vi "MGI Bezier Time.vi"(1 "t":sgl format="%.2f", 2 "First k":i32, 3 "Bezier Control Points[k]":sgl[](array[numeric]) format="%.4f") -> (0 "u":sgl format="%.2f")   [LabVIEW 2020]
doc: "Calculate a bezier 0..1 parameter from t. Actually uses a forward bezier instead of an inverse, so the endpoint times are first used to map t to a 0..1 parameter, then the bezier is calculated, then the endpoints are used to map the result back to 0..1.\n\nAuthored by David A. Moore\nsupport@mooregoodideas.com\nwww.mooregoodideas.com\n\nCopyright (c) 2010, Moore Good Ideas, Inc.\n\nAll rights reserved.\n\nRedistribution and use in source and binary forms, with or without modification, are permitted provided that the following conditions are met:\n\n * Redistributions of source code must retain the above copyright notice, this list of conditions and the following disclaimer.\n * Redistributions in binary form must reproduce the above copyright notice, this list of conditions and the following disclaimer in the documentation and/or other materials provided with the distribution.\n * Neither the name of Moore Good Ideas, Inc. nor the names of its contributors may be used to endorse or promote products derived from this software without specific prior written permission.\n\nTHIS SOFTWARE IS PROVIDED BY THE COPYRIGHT HOLDERS AND CONTRIBUTORS \"AS IS\" AND ANY EXPRESS OR IMPLIED WARRANTIES, INCLUDING, BUT NOT LIMITED TO, THE IMPLIED WARRANTIES OF MERCHANTABILITY AND FITNESS FOR A PARTICULAR PURPOSE ARE DISCLAIMED. IN NO EVENT SHALL THE COPYRIGHT OWNER OR CONTRIBUTORS BE LIABLE FOR ANY DIRECT, INDIRECT, INCIDENTAL, SPECIAL, EXEMPLARY, OR CONSEQUENTIAL DAMAGES (INCLUDING, BUT NOT LIMITED TO, PROCUREMENT OF SUBSTITUTE GOODS OR SERVICES; LOSS OF USE, DATA, OR PROFITS; OR BUSINESS INTERRUPTION) HOWEVER CAUSED AND ON ANY THEORY OF LIABILITY, WHETHER IN CONTRACT, STRICT LIABILITY, OR TORT (INCLUDING NEGLIGENCE OR OTHERWISE) ARISING IN ANY WAY OUT OF THE USE OF THIS SOFTWARE, EVEN IF ADVISED OF THE POSSIBILITY OF SUCH DAMAGE."
uses:
  <userlib>/_MGI/Bezier/MGI Bezier Weights/MGI Bezier Weights (SGL).vi
panel:
  # "k"
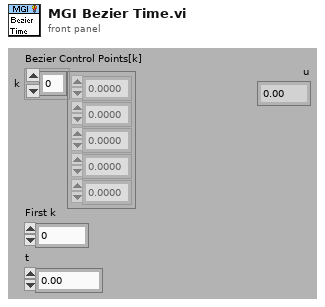
[diagram p1: front panel]
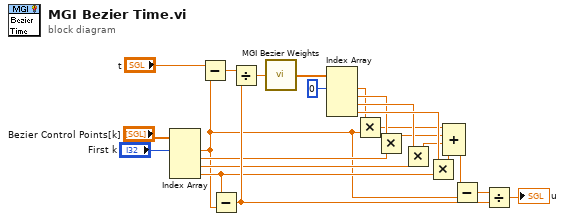
[diagram p0: block diagram]
diagram:
  n1 = Index Array(array="Bezier Control Points[k]", index #1="First k") -> (element #1=w3:sgl, element #2=w11:sgl, element #3=w13:sgl, element #4=w14:sgl)  [unwired: 3 in]
  n2 = Subtract(x="t", y=w3) -> (x-y=w19:sgl)
  n3 = Subtract(x=w14, y=w3) -> (x-y=w18:sgl)
  n4 = Divide(x=w19, y=w18) -> (x/y=w17:sgl)
  n5 = call-poly <userlib>:"MGI Bezier Weights.vi"("u"=w17) -> ("Bezier Weights"=w21:sgl[])
  n6 = Index Array(array=w21, index #1=0 ("Index")) -> (element #1=w9:sgl, element #2=w10:sgl, element #3=w12:sgl, element #4=w15:sgl)  [unwired: 3 in]
  n7 = Multiply(x=w9, y=w3) -> (x*y=w7:sgl)
  n8 = Multiply(x=w10, y=w11) -> (x*y=w6:sgl)
  n9 = Multiply(x=w12, y=w13) -> (x*y=w5:sgl)
  n10 = Multiply(x=w15, y=w14) -> (x*y=w8:sgl)
  n11 = Compound Arithmetic op=ADD(w7, w6, w5, w8) -> (w4:sgl)
  n12 = Subtract(x=w4, y=w3) -> (x-y=w2:sgl)
  n13 = Divide(x=w2, y=w18) -> (x/y=→"u":sgl)
